vi "dB.vi"(8 "error in (no error)":errorcluster, 9 "Magnitude":cluster{"f0":dbl, "df":dbl, "Mag H(w)":dbl[]}) -> (0 "error out":errorcluster, 1 "Magnitude [dB]":cluster{"f0":dbl, "df":dbl, "Mag H(w)":dbl[]})   [LabVIEW 2019]
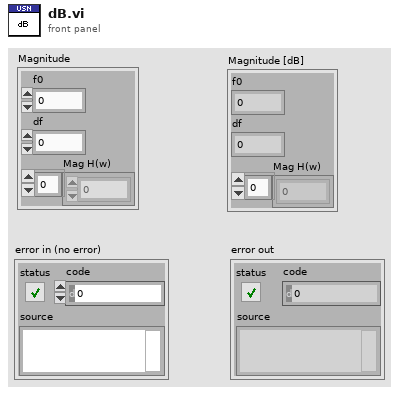
[diagram p1: front panel]
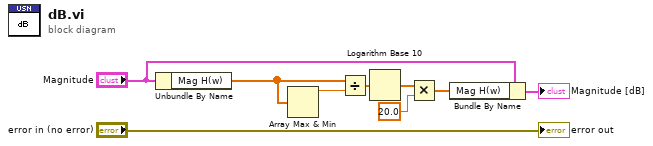
[diagram p0: block diagram]
diagram:
  n1 = Unbundle By Name("Magnitude") -> ("Mag H(w)"=w8:dbl[])
  n2 = Array Max & Min(array=w8) -> (max value=w9:dbl)  [unwired: 3 out]
  n3 = Divide(x=w8, y=w9) -> (x/y=w3:dbl[])
  n4 = Logarithm Base 10(1:w3) -> (0:w4:dbl[])
  n5 = Multiply(x=w4, y=20.0 ("Numeric")) -> (x*y=w6:dbl[])
  n6 = Bundle By Name(cluster="Magnitude", "Mag H(w)"=w6) -> (→"Magnitude [dB]":cluster{"f0":dbl, "df":dbl, "Mag H(w)":dbl[]})
  "error out" <- "error in (no error)"
